vi "Ins.KH7008.setAllChannels.vi"(8 "error in (no error)":errorcluster, 10 "allChannelProperties":T1 {"channel" min=1 max=8 step=1}, 11 "Inst.Krohn-Hite-7008 in":refnum<class "Inst.Krohn-Hite-7008.lvclass">) -> (0 "error out":errorcluster, 3 "Inst.Krohn-Hite-7008 out":refnum<class "Inst.Krohn-Hite-7008.lvclass">)   [LabVIEW 2019, in "Inst.Krohn-Hite-7008.lvclass"]
uses:
  Inst.Krohn-Hite-7008.lvclass
  KH7008/typedefs/allChannelProperties--Array.ctl
  KH7008/typedefs/channelProperties--Cluster.ctl
  KH7008/typedefs/channel--numeric.ctl
  KH7008/typedefs/gain--enum.ctl
  KH7008/typedefs/Input--Enum.ctl
  KH7008/typedefs/shunt--enum.ctl
  KH7008/typedefs/couple--Enum.ctl
  KH7008/typedefs/Filter--Enum.ctl
  Typedefs/setAllChannelsRequest--Cluster.ctl
  KH7008/KH7008.lvlib
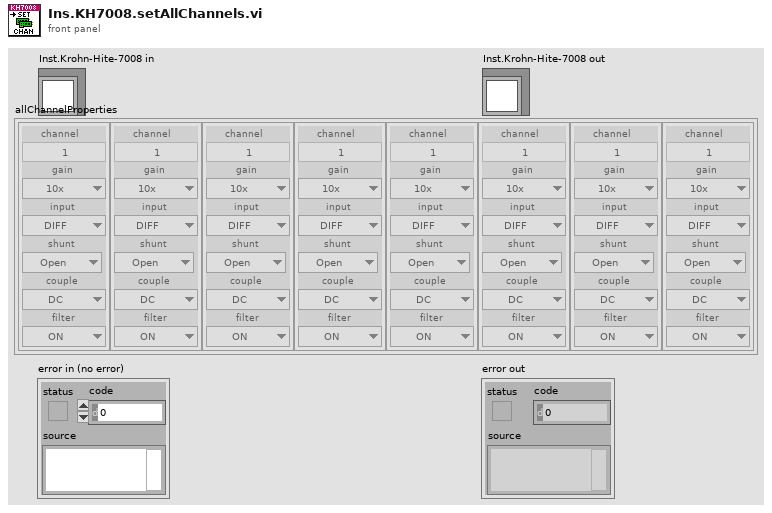
[diagram p1: front panel]
types:
  T1 = typedef "KH7008.lvlib/allChannelProperties--Array.ctl" = T2[]
  T2 = typedef "KH7008.lvlib/channelProperties--Cluster.ctl" = cluster{"channel":T3, "gain":T4, "input":T5, "shunt":T6, "couple":T7, "filter":T8}
  T3 = typedef "KH7008.lvlib/channel--numeric.ctl" = u16
  T4 = typedef "KH7008.lvlib/gain--enum.ctl" = enum16{"1x", "10x", "100x", "1000x"}
  T5 = typedef "KH7008.lvlib/input--enum.ctl" = enum16{"OFF", "SE+", "SE-", "DIFF"}
  T6 = typedef "KH7008.lvlib/shunt--enum.ctl" = enum16{"Open", "50", "500", "5k", "50k", "10M"}
  T7 = typedef "KH7008.lvlib/couple--enum.ctl" = enum16{"AC", "DC"}
  T8 = typedef "KH7008.lvlib/filter--enum.ctl" = enum16{"OFF", "ON"}
  T9 = typedef "Inst.Krohn-Hite-7008.lvclass/setAllChannelsRequest--Cluster.ctl" = cluster{"allChannelProperties":T1}
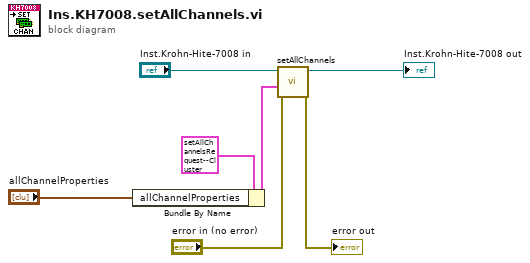
[diagram p0: block diagram]
diagram:
  n1 = Bundle By Name(cluster=T9 {"allChannelProperties"=[{"channel"=1, "gain"=enum."10x", "input"=enum."OFF", "shunt"=enum."10M", "couple"=enum."AC", "filter"=enum."OFF"}, {"channel"=2, "gain"=enum."10x", "input"=enum."OFF", "shunt"=enum."10M", "couple"=enum."AC", "filter"=enum."OFF"}, {"channel"=3, "gain"=enum."10x", "input"=enum."OFF", "shunt"=enum."10M", "couple"=enum."AC", "filter"=enum."OFF"}, {"channel"=4, "gain"=enum."10x", "input"=enum."OFF", "shunt"=enum."10M", "couple"=enum."AC", "filter"=enum."OFF"}, {"channel"=5, "gain"=enum."10x", "input"=enum."OFF", "shunt"=enum."10M", "couple"=enum."AC", "filter"=enum."OFF"}, {"channel"=6, "gain"=enum."10x", "input"=enum."OFF", "shunt"=enum."10M", "couple"=enum."AC", "filter"=enum."OFF"}, {"channel"=7, "gain"=enum."10x", "input"=enum."OFF", "shunt"=enum."10M", "couple"=enum."AC", "filter"=enum."OFF"}, {"channel"=7, "gain"=enum."10x", "input"=enum."OFF", "shunt"=enum."10M", "couple"=enum."AC", "filter"=enum."OFF"}]} ("setAllChannelsRequest"), "allChannelProperties"="allChannelProperties") -> (w2:T9)
  n2 = call-dynamic "setAllChannels.vi"("error in (no error)"="error in (no error)", "allChannelProperties"=w2, "Inst.Krohn-Hite-7008 in"="Inst.Krohn-Hite-7008 in") -> ("error out"=→"error out":errorcluster, "Inst.Krohn-Hite-7008 out"=→"Inst.Krohn-Hite-7008 out":refnum<class "Inst.Krohn-Hite-7008.lvclass">)  [unwired: 7 in]
